vi "Go Down (Loaded).vi"(6 "Skip Load?":bool, 7 "Model Name":T2, 8 "Error In":errorcluster, 9 "Intialize?":bool=TRUE, 10 "Inputs":T3) -> (0 "error out":errorcluster, 1 "Completed":bool, 3 "Results":T1, 4 "Status":cluster{"Status":string, "Elapsed Time":dbl}, 5 "Array":dbl[][](array[numeric]))   [LabVIEW 2017]
doc: "Changelog:\n\n------------\nv0.2:\n- Bypass sensor 1 for all front\n\n\nv0.1:\n- Start Travel time taken from when the start moving command is given (previous state)\n- Total travel time is taken until the movement is stopped"
uses:
  controls/All Inputs.ctl
  controls/SACB DI.ctl
  controls/Model Name.ctl
  controls/Go Down (Loaded).ctl
  controls/FGV DO.ctl
panel:
  in  "Stall Time (ms)":u32=200
  in  "Delay (for Rest)":u32=500
  in  "Timeout (ms)":u32=15000
  # "Inputs"
  # "Variables"
  # "Outputs"
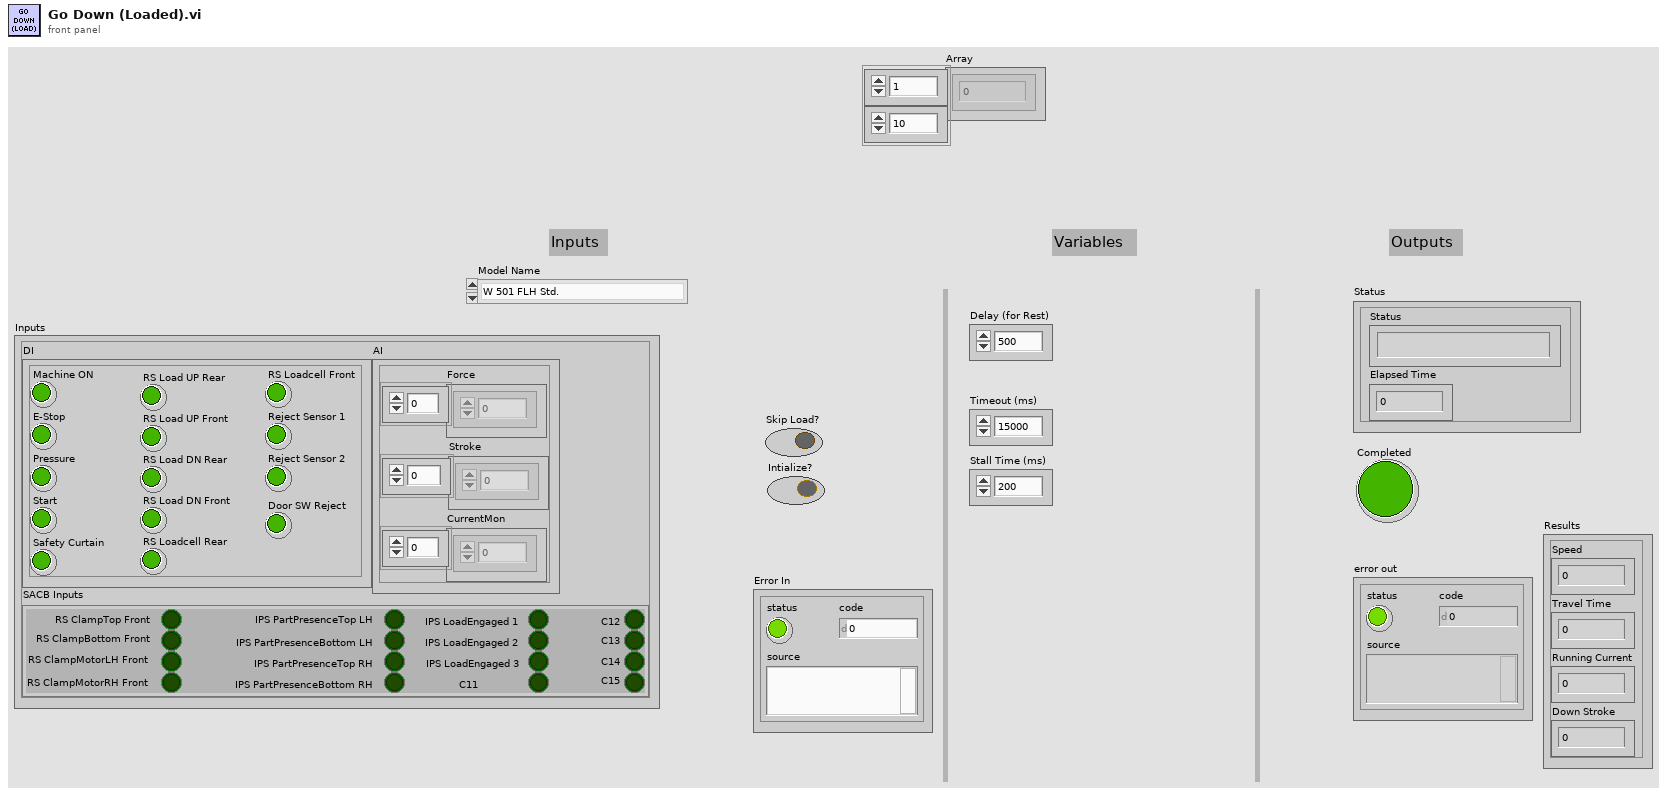
[diagram p1: front panel]
types:
  T1 = cluster{"Speed":dbl, "Travel Time":dbl, "Running Current":dbl, "Down Stroke":dbl}
  T2 = typedef "Model Name.ctl" = enum16{"W 501 FLH Std.", "W 501 FRH Std.", "W 601 FR RH Std", "W 601 FR LH Std", "W 601 RR RH Std", "W 601 RR LH Std", "W 601 FR RH AP", "W 601 FR LH AP", "W 601 RR RH AP", "W 601 RR LH AP"}
  T3 = typedef "All Inputs.ctl" = cluster{"DI":cluster{"Machine ON":bool, "E-Stop":bool, "Pressure":bool, "Start":bool, "Safety Curtain":bool, "RS Load UP Rear":bool, "RS Load UP Front":bool, "RS Load DN Rear":bool, "RS Load DN Front":bool, "RS Loadcell Rear":bool, "RS Loadcell Front":bool, "Reject Sensor 1":bool, "Reject Sensor 2":bool, "Door SW Reject":bool}, "AI":cluster{"Force":dbl[], "Stroke":dbl[], "CurrentMon":dbl[]}, "SACB Inputs":T4}
  T4 = typedef "SACB DI.ctl" = cluster{"RS ClampTop Front":bool, "RS ClampBottom Front":bool, "RS ClampMotorLH Front":bool, "RS ClampMotorRH Front":bool, "IPS PartPresenceTop LH":bool, "IPS PartPresenceBottom LH":bool, "IPS PartPresenceTop RH":bool, "IPS PartPresenceBottom RH":bool, "IPS LoadEngaged 1":bool, "IPS LoadEngaged 2":bool, "IPS LoadEngaged 3":bool, "C11":bool, "C12":bool, "C13":bool, "C14":bool, "C15":bool}
  T5 = typedef "Go Down (Loaded).ctl" = enum16{"Initialize", "Set Loading", "Check Top Position", "Go Down", "Wait for Stall", "Turn Off Supply", "Wait for Rest", "Done", "Error"}
  T6 = typedef "FGV DO.ctl" = enum16{"Initialize", "Start Task", "Clamping", "Load CYL", "Contactors", "Loadcell CYL", "BSL", "Read DO", "Clear Tasks", "Clear Task"}
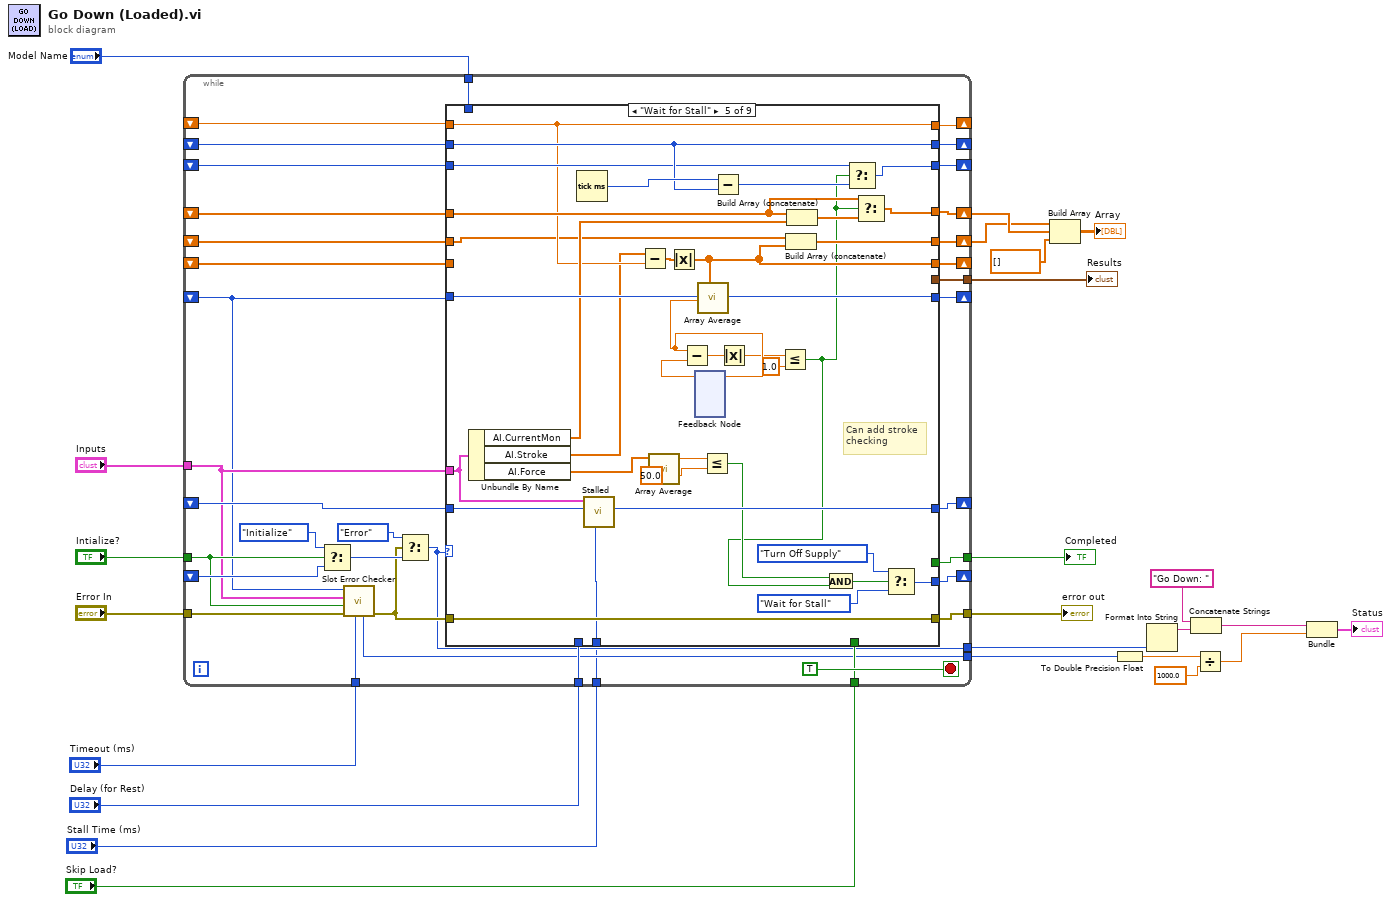
[diagram p0: block diagram]
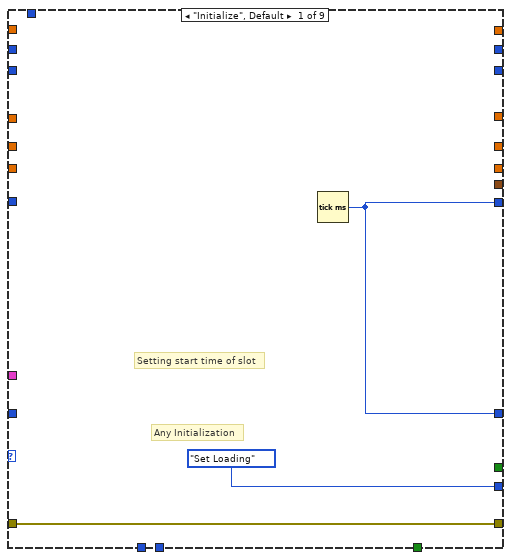
[diagram p2: hidden frame]
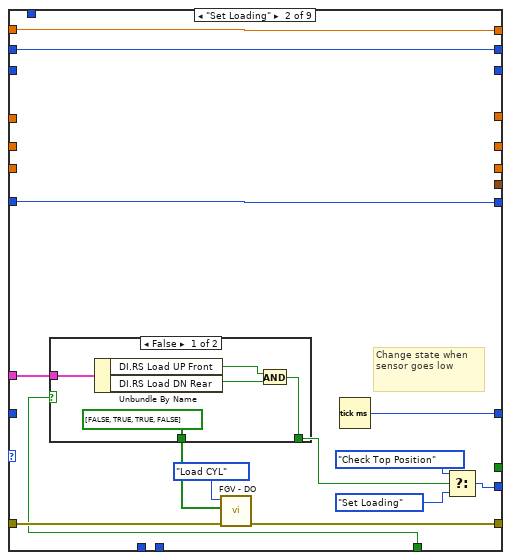
[diagram p3: hidden frame]
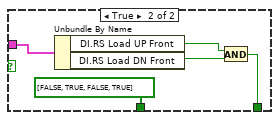
[diagram p4: hidden frame]
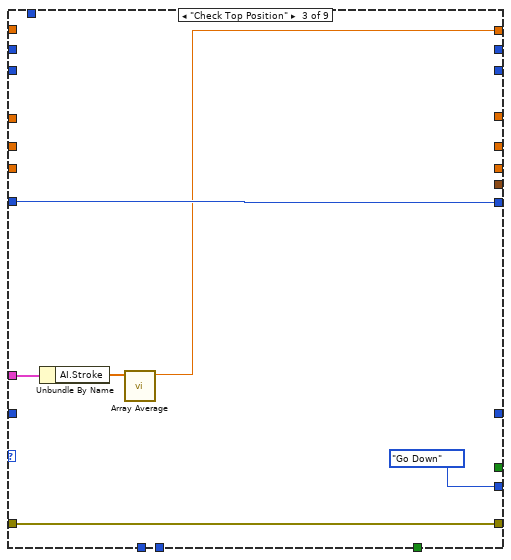
[diagram p5: hidden frame]
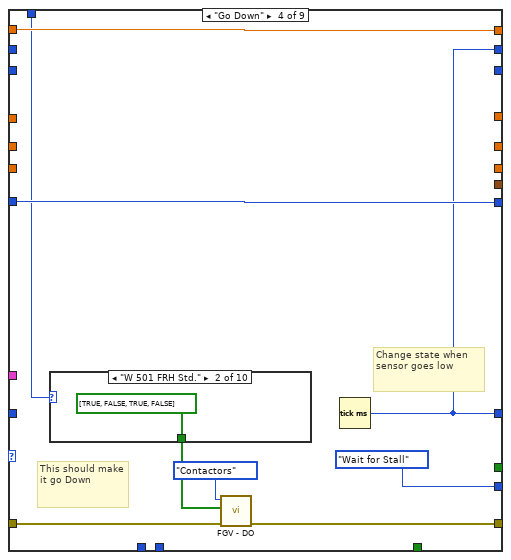
[diagram p6: hidden frame]
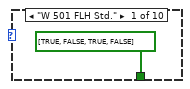
[diagram p7: hidden frame]
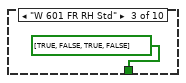
[diagram p8: hidden frame]
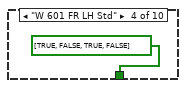
[diagram p9: hidden frame]
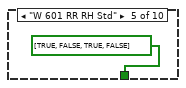
[diagram p10: hidden frame]
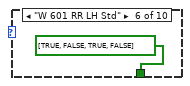
[diagram p11: hidden frame]
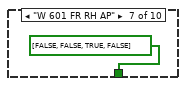
[diagram p12: hidden frame]
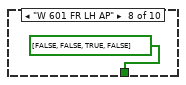
[diagram p13: hidden frame]
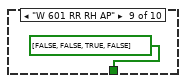
[diagram p14: hidden frame]
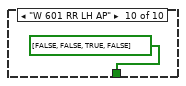
[diagram p15: hidden frame]
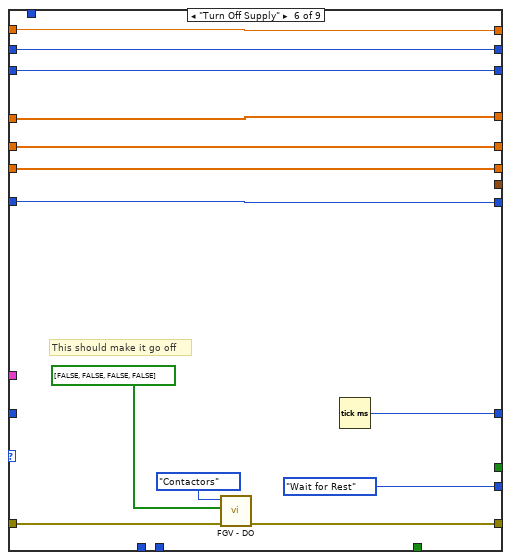
[diagram p16: hidden frame]
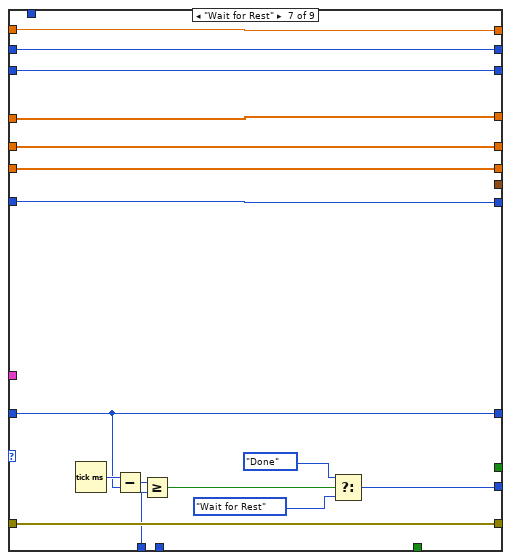
[diagram p17: hidden frame]
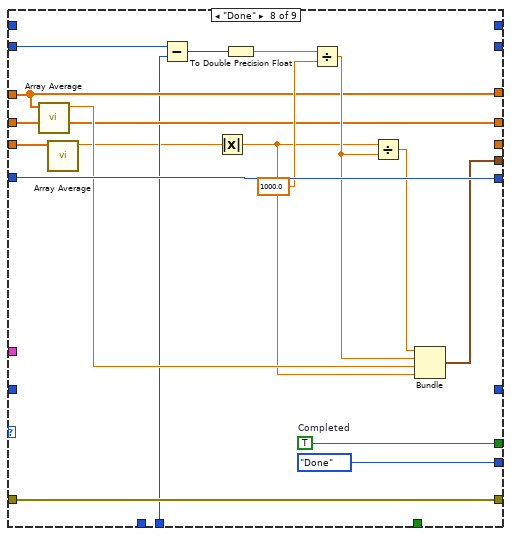
[diagram p18: hidden frame]
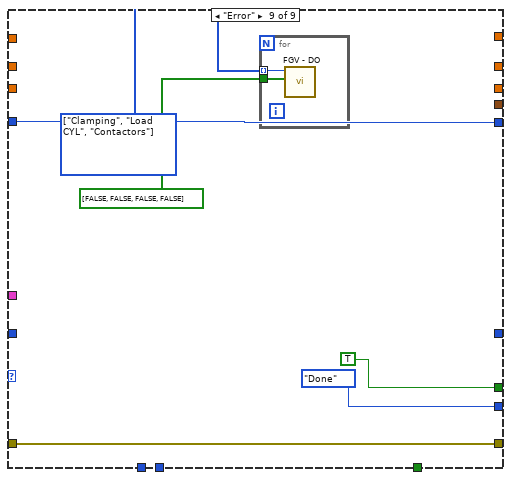
[diagram p19: hidden frame]
diagram:
  n1 = while {
    tunnel: "Intialize?" -> [w50]
    shift-right: [w57] -> _
    shift-left: _ -> [w59]
    shift-right: [w56] -> _
    shift-left: _ -> [w55]
    tunnel: "Error In" -> [w51]
    tunnel: [w54] -> w24
    tunnel: [w53] -> w23
    tunnel: "Inputs" -> [w49]
    shift-right: [w52] -> _
    shift-left: _ -> [w48]
    tunnel: "Delay (for Rest)" -> [w44]
    tunnel: "Timeout (ms)" -> [w43]
    tunnel: "Model Name" -> [w42]
    shift-right: [w41] -> _
    shift-left: _ -> [w40]
    shift-right: [w39] -> _
    shift-left: _ -> [w38]
    shift-right: [w37] -> w5
    shift-left: _ -> [w36]
    shift-right: [w35] -> _
    shift-left: _ -> [w34]
    shift-right: [w33] -> _
    shift-left: _ -> [w32]
    tunnel: [w31] -> w6
    tunnel: "Skip Load?" -> [w30]
    tunnel: [w29] -> w8
    tunnel: [w28] -> w7
    shift-right: [w27] -> w3
    shift-left: _ -> [w26]
    tunnel: "Stall Time (ms)" -> [w25]
    stop <- TRUE stop-if-true
    n2 = Select(t=Go_Down_(Loaded)."Initialize", s=w50, f=w59) -> (s? t:f=w47:T5)
    n3 = call "Slot Error Checker.vi"("Timeout (ms)"=w43, "error in (no error)"=w51, "Intialize?"=w50, "Inputs"=w49, "start time"=w48) -> ("error out"=w46:errorcluster, "Slot Time"=w29:u32)  [unwired: 4 in, 1 out]
    n4 = Select(t=Go_Down_(Loaded)."Error", s=w46, f=w47) -> (s? t:f=w28:T5)
    n5 = case shown="\"Wait for Stall\"" w28 {
      tunnel: [Go_Down_(Loaded)."Set Loading" w71 Go_Down_(Loaded)."Go Down" Go_Down_(Loaded)."Wait for Stall" w141 Go_Down_(Loaded)."Wait for Rest" w173 Go_Down_(Loaded)."Done" Go_Down_(Loaded)."Done"] -> w57
      tunnel: [w61 w68 _ w94 w144 w156 w175 _ _] -> w56
      tunnel: w55 -> [_ _ _ _ w145 _ w175 _ _]
      tunnel: w46 -> [w62 w77 w92 w102 w146 w160 w171 w193 w200]
      tunnel: [w62 w76 w92 w101 w146 w159 w171 w193 w200] -> w54
      tunnel: [_ _ _ _ _ _ _ w192 TRUE ("Completed")] -> w53
      tunnel: w49 -> [_ w65 w90 _ w140 _ _ _ _]
      tunnel: [w61 w73 w93 w98 w147 w155 w168 w191 w197] -> w52
      tunnel: w48 -> [_ w73 w93 w98 w147 w155 w168 w191 w197]
      tunnel: w44 -> [_ _ _ _ _ _ w167 _ _]
      tunnel: w42 -> [_ _ _ w96 _ _ _ _ _]
      tunnel: [_ w72 w88 w97 w124 w151 w162 _ _] -> w41
      tunnel: w40 -> [_ w72 _ w97 w124 w151 w162 _ _]
      tunnel: [_ w67 _ w94 w136 w152 w163 _ _] -> w39
      tunnel: w38 -> [_ w67 _ _ w136 w152 w163 _ _]
      tunnel: [_ _ _ _ w139 w154 w165 w183 _] -> w37
      tunnel: w36 -> [_ _ _ _ w126 w154 w165 w183 _]
      tunnel: [_ _ _ _ w135 w153 w164 _ _] -> w35
      tunnel: w34 -> [_ _ _ _ w134 w153 w164 w190 _]
      tunnel: [_ _ _ _ w117 w150 w166 _ _] -> w33
      tunnel: w32 -> [_ _ _ _ _ w150 w166 w180 _]
      tunnel: [_ _ _ _ _ _ _ w184 _] -> w31
      tunnel: w30 -> [_ w66 _ _ _ _ _ _ _]
      tunnel: [_ _ _ _ w131 w148 w161 w182 _] -> w27
      tunnel: w26 -> [_ _ _ _ w123 w148 w161 w182 _]
      tunnel: w25 -> [_ _ _ _ w125 _ _ w178 _]
      frame "Initialize", Default {
        # "Setting start time of slot"
        # "Any Initialization"
        n6 = Tick Count (ms)() -> (millisecond timer value=w61:u32)
      }
      frame "Set Loading" {
        # "Change state when sensor goes low"
        n7 = case shown="False" w66 {
          tunnel: [bool[] [FALSE, TRUE, TRUE, FALSE] ("Digital Outs") bool[] [FALSE, TRUE, FALSE, TRUE] ("Digital Outs")] -> w74
          tunnel: w65 -> [w79 w86]
          tunnel: [w78 w83] -> w64
          frame False {
            n8 = Unbundle By Name(w79) -> ("DI.RS Load UP Front"=w81:bool, "DI.RS Load DN Rear"=w80:bool)
            n9 = And(x=w81, y=w80) -> (x .and. y?=w78:bool)
          }
          frame True {
            n10 = Unbundle By Name(w86) -> ("DI.RS Load UP Front"=w85:bool, "DI.RS Load DN Front"=w84:bool)
            n11 = And(x=w85, y=w84) -> (x .and. y?=w83:bool)
          }
        }
        n12 = call "FGV - DO.vi"("error in"=w77, "Digital Outs"=w74, "State"=FGV_DO."Load CYL") -> ("error out"=w76:errorcluster)  [unwired: 7 in, 1 out]
        n13 = Tick Count (ms)() -> (millisecond timer value=w68:u32)
        n14 = Select(t=Go_Down_(Loaded)."Check Top Position", s=w64, f=Go_Down_(Loaded)."Set Loading") -> (s? t:f=w71:T5)
      }
      frame "Check Top Position" {
        n15 = Unbundle By Name(w90) -> ("AI.Stroke"=w89:dbl[])
        n16 = call "Array Average.vi"("data"=w89) -> ("Numeric"=w88:dbl)  [unwired: 10 in]
      }
      frame "Go Down" {
        # "Change state when sensor goes low"
        # "This should make it go Down"
        n17 = case shown="\"W 501 FRH Std.\"" w96 {
          tunnel: [bool[] [TRUE, FALSE, TRUE, FALSE] ("Digital Outs") bool[] [TRUE, FALSE, TRUE, FALSE] ("Digital Outs") bool[] [TRUE, FALSE, TRUE, FALSE] ("Digital Outs") bool[] [TRUE, FALSE, TRUE, FALSE] ("Digital Outs") bool[] [TRUE, FALSE, TRUE, FALSE] ("Digital Outs") bool[] [TRUE, FALSE, TRUE, FALSE] ("Digital Outs") bool[] [FALSE, FALSE, TRUE, FALSE] ("Digital Outs") bool[] [FALSE, FALSE, TRUE, FALSE] ("Digital Outs") bool[] [FALSE, FALSE, TRUE, FALSE] ("Digital Outs") bool[] [FALSE, FALSE, TRUE, FALSE] ("Digital Outs")] -> w99
          frame "W 501 FLH Std." {
          }
          frame "W 501 FRH Std." {
          }
          frame "W 601 FR RH Std" {
          }
          frame "W 601 FR LH Std" {
          }
          frame "W 601 RR RH Std" {
          }
          frame "W 601 RR LH Std" {
          }
          frame "W 601 FR RH AP" {
          }
          frame "W 601 FR LH AP" {
          }
          frame "W 601 RR RH AP" {
          }
          frame "W 601 RR LH AP" {
          }
        }
        n18 = call "FGV - DO.vi"("error in"=w102, "Digital Outs"=w99, "State"=FGV_DO."Contactors") -> ("error out"=w101:errorcluster)  [unwired: 7 in, 1 out]
        n19 = Tick Count (ms)() -> (millisecond timer value=w94:u32)
      }
      frame "Wait for Stall" {
        # "Can add stroke checking"
        n20 = Unbundle By Name(w140) -> ("AI.CurrentMon"=w133:dbl[], "AI.Stroke"=w122:dbl[], "AI.Force"=w121:dbl[])
        n21 = Tick Count (ms)() -> (millisecond timer value=w137:u32)
        n22 = call "Stalled.vi"("Stall Time (ms)"=w125, "millisecond timer value in"=w145, "Inputs"=w140) -> ("millisecond timer value out"=w144:u32)  [unwired: 7 in, 1 out]
        n23 = Subtract(x=w122, y=w124) -> (x-y=w118:dbl[])
        n24 = call "Array Average.vi"("data"=w121) -> ("Numeric"=w127:dbl)  [unwired: 10 in]
        n25 = Absolute Value(x=w118) -> (abs(x)=w117:dbl[])
        n26 = feedback #1() -> (w119:dbl)  [unwired: 1 in]
        n27 = call "Array Average.vi"("data"=w117) -> ("Numeric"=w116:dbl)  [unwired: 10 in]
        n28 = Subtract(x=w116, y=w119) -> (x-y=w120:dbl)
        n29 = feedback-in #1(w116) -> ()
        n30 = Less Or Equal?(x=w127, y=50.0) -> (x <= y?=w129:bool)
        n31 = Subtract(x=w137, y=w136) -> (x-y=w132:u32)
        n32 = Absolute Value(x=w120) -> (abs(x)=w114:dbl)
        n33 = Less Or Equal?(x=w114, y=1.0) -> (x <= y?=w113:bool)
        n34 = Build Array (concatenate)(w123, w117) -> (w131:dbl[])
        n35 = Build Array (concatenate)(w126, w133) -> (w138:dbl[])
        n36 = And(x=w129, y=w113) -> (x .and. y?=w128:bool)
        n37 = Select(t=w134, s=w113, f=w132) -> (s? t:f=w135:u32)
        n38 = Select(t=w126, s=w113, f=w138) -> (s? t:f=w139:dbl[])
        n39 = Select(t=Go_Down_(Loaded)."Turn Off Supply", s=w128, f=Go_Down_(Loaded)."Wait for Stall") -> (s? t:f=w141:T5)
      }
      frame "Turn Off Supply" {
        # "This should make it go off"
        n40 = call "FGV - DO.vi"("error in"=w160, "Digital Outs"=bool[] [FALSE, FALSE, FALSE, FALSE], "State"=FGV_DO."Contactors") -> ("error out"=w159:errorcluster)  [unwired: 7 in, 1 out]
        n41 = Tick Count (ms)() -> (millisecond timer value=w156:u32)
      }
      frame "Wait for Rest" {
        n42 = Tick Count (ms)() -> (millisecond timer value=w176:u32)
        n43 = Subtract(x=w176, y=w175) -> (x-y=w174:u32)
        n44 = Greater Or Equal?(x=w174, y=w167) -> (x >= y?=w172:bool)
        n45 = Select(t=Go_Down_(Loaded)."Done", s=w172, f=Go_Down_(Loaded)."Wait for Rest") -> (s? t:f=w173:T5)
      }
      frame "Done" {
        w192 = TRUE  # Completed
        n46 = call "Array Average.vi"("data"=w183) -> ("Numeric"=w185:dbl)  [unwired: 10 in]
        n47 = call "Array Average.vi"("data"=w180) -> ("Numeric"=w177:dbl)  [unwired: 10 in]
        n48 = Subtract(x=w190, y=w178) -> (x-y=w179:u32)
        n49 = Absolute Value(x=w177) -> (abs(x)=w181:dbl)
        n50 = To Double Precision Float(number=w179) -> (double precision float=w188:dbl)
        n51 = Divide(x=w188, y=1000.0) -> (x/y=w186:dbl)
        n52 = Divide(x=w181, y=w186) -> (x/y=w187:dbl)
        n53 = Bundle(w187, w186, "Numeric"=w185, w181) -> (w184:cluster{dbl, dbl, "Numeric":dbl, dbl})  [unwired: 1 in]
      }
      frame "Error" {
        w195 = T6[] [enum."Clamping", enum."Load CYL", enum."Contactors"] items=["Initialize", "Start Task", "Clamping", "Load CYL", "Contactors", "Loadcell CYL", "BSL", "Read DO", "Clear Tasks", "Clear Task"]
        n54 = for {
          tunnel: w195 -> [w202] mode=indexing
          tunnel: bool[] [FALSE, FALSE, FALSE, FALSE] ("Digital Outs") -> [w201]
          n55 = call "FGV - DO.vi"("Digital Outs"=w201, "State"=w202) -> ()  [unwired: 8 in, 2 out]
        }
      }
    }
  }
  "error out" <- w24
  "Completed" <- w23
  "Results" <- w6
  n56 = Build Array(w3, w5, dbl[] [] ("element")) -> (→"Array":dbl[][])
  n57 = To Double Precision Float(number=w8) -> (double precision float=w13:dbl)
  n58 = Format Into String(w7) -> (resulting string=w15:string)  [unwired: 3 in, 1 out]
  n59 = Concatenate Strings("Go Down: ", w15) -> (w11:string)
  n60 = Divide(x=w13, y=1000.0) -> (x/y=w10:dbl)
  n61 = Bundle(w11, w10) -> (→"Status":cluster{string, dbl})  [unwired: 1 in]
